vi "InitAction.vi"(6 "InstrumentName":string, 7 "VisaRessIn":refnum<visa-resource-name>, 8 "error in (no error)":errorcluster caption="entrée d'erreur (pas d'erreur)", 9 "FirstClassInst":bool, 10 "Function":string, 11 "GenData In":refnum<class "KlingerMotor.lvclass"> caption="DNL_LabVIEW Object in") -> (0 "error out":errorcluster caption="sortie d'erreur", 3 "GenData Out":refnum<class "KlingerMotor.lvclass"> caption="DNL_LabVIEW Object out")   [LabVIEW 2012, in "KlingerMotor.lvclass"]
uses:
  KlingerMotor.lvclass
  KlingerMotor_Func.ctl
  KlingerMotor.lvclass/KlingerMotor.ctl
panel:
  in  "DefaultDev_Func":T1
  out "VisaRessOut":refnum<visa-resource-name>
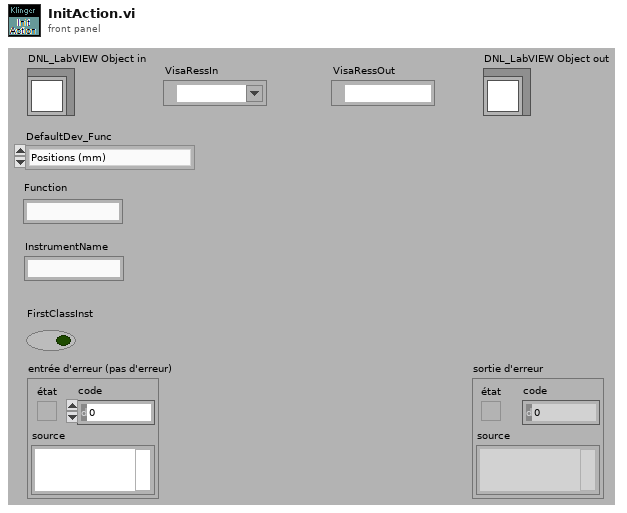
[diagram p1: front panel]
types:
  T1 = typedef "KlingerMotor.lvclass/KlingerMotor_Func.ctl" = enum16{"Positions (mm)", "Position (ps)", "ReadWPos (ps)", "ReadWPos (mm)", "ReadZPos (ps)", "ReadZPos (mm)"}
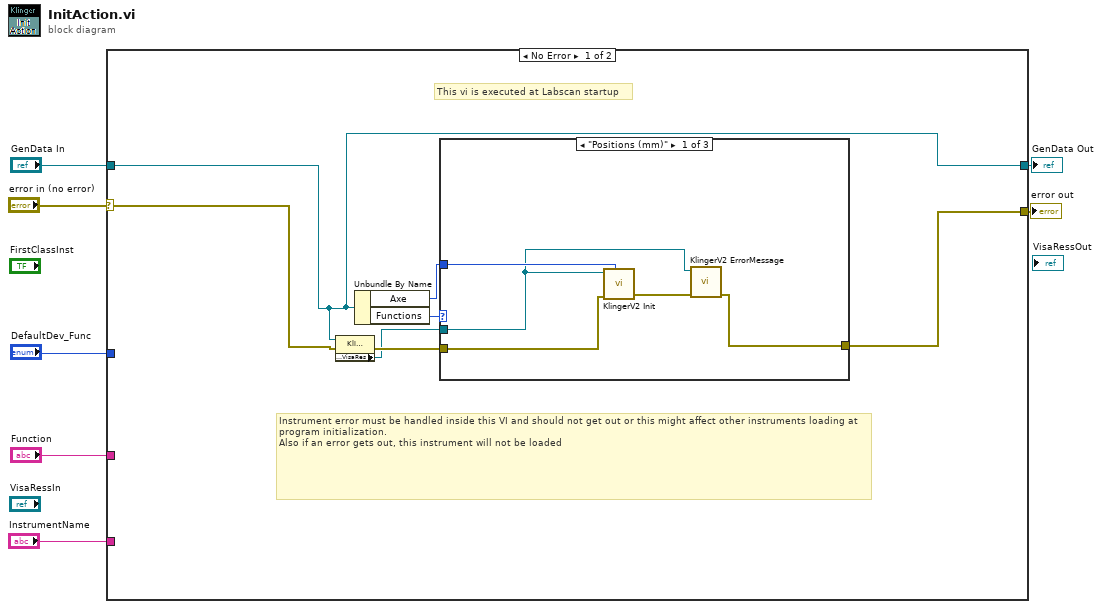
[diagram p0: block diagram]
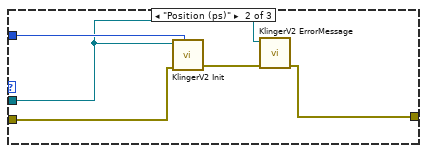
[diagram p2: hidden frame]
diagram:
  n1 = case shown="No Error" "error in (no error)" {
    selector: "error in (no error)" -> [w10 w27]
    tunnel: [w12 w27] -> w6
    tunnel: "GenData In" -> [w11 w26]
    tunnel: [w11 w26] -> w4
    tunnel: "DefaultDev_Func" -> [_ _]
    tunnel: "Function" -> [_ _]
    tunnel: "InstrumentName" -> [_ _]
    frame No Error {
      # "This vi is executed at Labscan startup"
      # "Instrument error must be handled inside this VI and should not get out or this might affect other instruments loading at program initialization.\nAlso if an error gets out, this instrument will not be loaded"
      n2 = property class="KlingerMotor.lvclass"(reference=w11, error in=w10) -> (error out=w9:errorcluster, "Accessor:VisaRes"=w8:refnum<visa-resource-name>)  [unwired: 1 out]
      n3 = Unbundle By Name(w11) -> ("Axe"=w13:u8, "Functions"=w14:T1)
      n4 = case shown="\"Positions (mm)\"" w14 {
        tunnel: w13 -> [w19 w24 _]
        tunnel: w9 -> [w18 w23 w25]
        tunnel: [w15 w20 w25] -> w12
        tunnel: w8 -> [w16 w21 _]
        frame "Positions (mm)" {
          n5 = call <userlib>:"KlingerV2 Init.vi"("VISA_Res"=w16, "error in"=w18, "Axe"=w19) -> ("error out"=w17:errorcluster)  [unwired: 2 in, 2 out]
          n6 = call <userlib>:"KlingerV2 ErrorMessage.vi"("error in (no error)"=w17, "VisaRes"=w16) -> ("error out"=w15:errorcluster)  [unwired: 8 in, 1 out]
        }
        frame "Position (ps)" {
          n7 = call <userlib>:"KlingerV2 Init.vi"("VISA_Res"=w21, "error in"=w23, "Axe"=w24) -> ("error out"=w22:errorcluster)  [unwired: 2 in, 2 out]
          n8 = call <userlib>:"KlingerV2 ErrorMessage.vi"("error in (no error)"=w22, "VisaRes"=w21) -> ("error out"=w20:errorcluster)  [unwired: 8 in, 1 out]
        }
        frame Default {
        }
      }
    }
    frame Error {
    }
  }
  "error out" <- w6
  "GenData Out" <- w4
